vi "Get Labels on Port.vi"(8 "error in":errorcluster, 11 "port ref":T1 format="%.0x") -> (0 "error out":errorcluster, 1 "labels properties":T2[](array[typedef]), 2 "label references":T1[](array[typedef]) format="%.0x", 3 "port ref out":T1 format="%.0x")   [LabVIEW 2020, in "ARINC 429 Scripting.lvlib"]
uses:
  ARINC 429 Scripting.lvlib
  <vilib>/NI VeriStand/Custom Device API/Custom Device Item Ref.ctl
  Shared/Label Properties.ctl
  Ballard/Constants.vi
  <vilib>/NI VeriStand/Custom Device Tools/Custom Device Utility Library/NI VeriStand - Search for All Items by GUID.vi
  <vilib>/NI VeriStand/Custom Device Tools/Custom Device Utility Library/Custom Device Utility Library.lvlib
  Ballard/Ballard ARINC 429 Scripting.lvlib
  <vilib>/NI VeriStand/Custom Device API/Custom Device API.lvlib
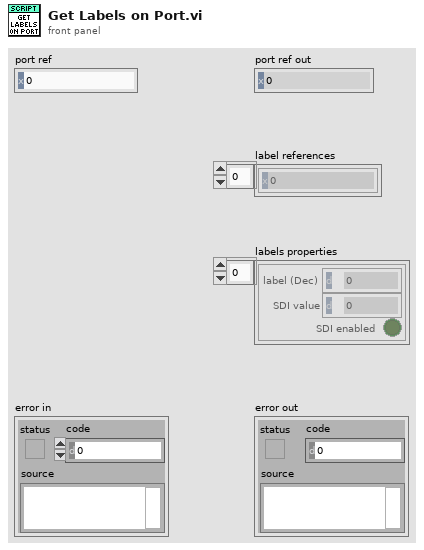
[diagram p1: front panel]
types:
  T1 = typedef "Custom Device API.lvlib/Custom Device Item Ref.ctl" = u64
  T2 = typedef "Label Properties.ctl" = cluster{"label (Dec)":u32, "SDI value":u8, "SDI enabled":bool}
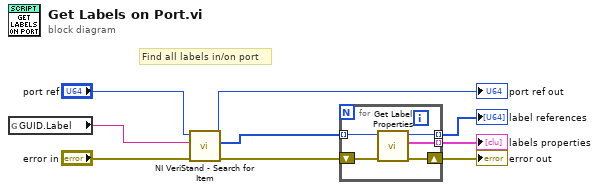
[diagram p0: block diagram]
diagram:
  # "Find all labels in/on port"
  n1 = global read "Constants.vi" "GUID.Label"() -> (w7:string)
  n2 = call-poly <vilib>:"NI VeriStand - Search for Item.vi"("error in"="error in", "Item GUID"=w7, "Section Ref in"="port ref") -> ("error out"=w2:errorcluster, "Item Refs"=w4:T1[], "Section Ref out"=→"port ref out":T1)  [unwired: 5 in, 1 out]
  n3 = for {
    shift-right: [w11] -> w9
    shift-left: w2 -> [w14]
    tunnel: w4 -> [w13] mode=indexing
    tunnel: [w12] -> w8 mode=indexing
    tunnel: [w10] -> w1 mode=indexing
    n4 = call "Get Label Properties.vi"("error in"=w14, "label ref in"=w13) -> ("error out"=w11:errorcluster, "label properties"=w10:T2, "label ref out"=w12:T1)  [unwired: 7 in]
  }
  "error out" <- w9
  "labels properties" <- w1
  "label references" <- w8
